vi "GetOrMakeSpecializedEditor.vi"() -> ()   [LabVIEW 2020, in "FlexBlocks.lvlib"]
uses:
  FlexBlocks.lvlib
panel:
  in  "Type":variant
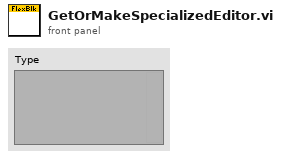
[diagram p1: front panel]
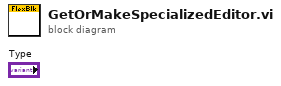
[diagram p0: block diagram]
diagram:
